vi "UDP Send and Receive (repeat on error) - DBL.vi"(7 "timeout ms (100)":i32=100, 8 "error in (no error)":errorcluster, 9 "DBL Command & Param":T1, 10 "IP":string, 11 "connection ID in":refnum<k16>) -> (0 "error out":errorcluster, 2 "DBL Param out":dbl, 3 "connection ID out":refnum<k16>)   [LabVIEW 2016, in "SMD-7615.lvlib" / "eSCL.lvlib"]
doc: "AC - Acceleration Rate\nSets or requests the acceleration rate used in point-to-point move commands in rev/sec/sec."
uses:
  eSCL.lvlib
  DBL Command and Param.ctl
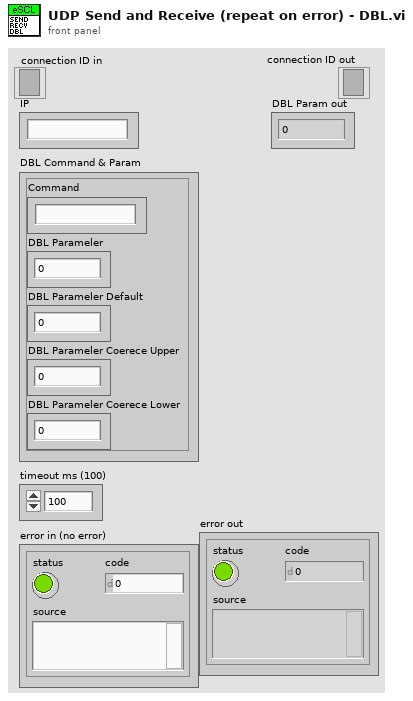
[diagram p1: front panel]
types:
  T1 = typedef "SMD-7615.lvlib/eSCL.lvlib/DBL Command and Param.ctl" = cluster{"Command":string, "DBL Parameler":dbl, "DBL Parameler Default":dbl, "DBL Parameler Coerece Upper":dbl, "DBL Parameler Coerece Lower":dbl}
  T2 = typedef "SMD-7615.lvlib/eSCL.lvlib/UDP Received Data.ctl" = cluster{"Received String":string, "eSCL Cmd":string, "Data":string}
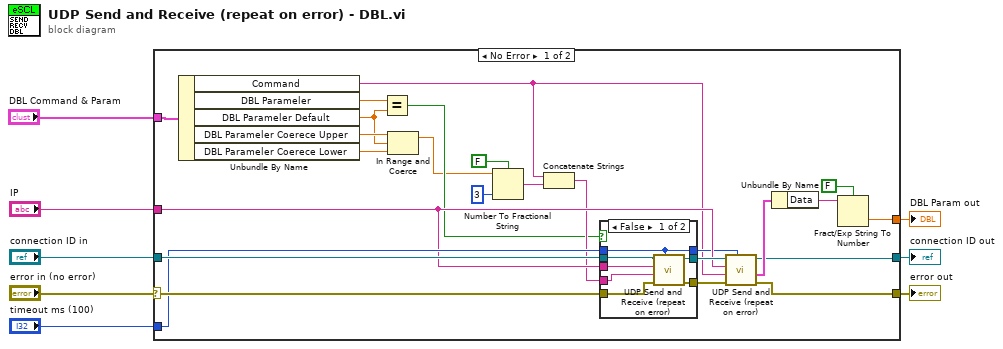
[diagram p0: block diagram]
diagram:
  n1 = case shown="No Error" "error in (no error)" {
    selector: "error in (no error)" -> [w33 w44]
    tunnel: "connection ID in" -> [w32 w45]
    tunnel: [w20 w45] -> w6
    tunnel: [w19 w44] -> w5
    tunnel: "IP" -> [w22 _]
    tunnel: "timeout ms (100)" -> [w23 _]
    tunnel: [w30 _] -> w2
    tunnel: "DBL Command & Param" -> [w14 _]
    frame No Error {
      n2 = Unbundle By Name(w14) -> ("Command"=w9:string, "DBL Parameler"=w13:dbl, "DBL Parameler Default"=w10:dbl, "DBL Parameler Coerece Upper"=w12:dbl, "DBL Parameler Coerece Lower"=w11:dbl)
      n3 = Equal?(x=w13, y=w10) -> (x = y?=w16:bool)
      n4 = In Range and Coerce(upper limit=w12, x=w10, lower limit=w11) -> (coerced(x)=w15:dbl)  [unwired: 1 out]
      n5 = Number To Fractional String(use system decimal point (T)=FALSE, number=w15, precision (6)=i16 3) -> (F-format string=w26:string)  [unwired: 1 in]
      n6 = Concatenate Strings(w9, w26) -> (w18:string)
      n7 = case shown="False" w16 {
        tunnel: w33 -> [w40 w41]
        tunnel: w32 -> [w39 w43]
        tunnel: [w38 w41] -> w25
        tunnel: [w37 w43] -> w24
        tunnel: w23 -> [w34 w42]
        tunnel: w22 -> [w36 _]
        tunnel: w18 -> [w35 _]
        tunnel: [w34 w42] -> w17
        frame False {
          n8 = call "UDP Send and Receive (repeat on error).vi"("timeout ms (100)"=w34, "error in (no error)"=w40, "Data"=w35, "IP"=w36, "connection ID in"=w39) -> ("error out"=w38:errorcluster, "connection ID out"=w37:refnum<k16>)  [unwired: 3 in, 2 out]
        }
        frame True {
        }
      }
      n9 = call "UDP Send and Receive (repeat on error).vi"("timeout ms (100)"=w17, "error in (no error)"=w25, "Data"=w9, "IP"=w22, "connection ID in"=w24) -> ("error out"=w19:errorcluster, "Received Data"=w21:T2, "connection ID out"=w20:refnum<k16>)  [unwired: 3 in, 1 out]
      n10 = Unbundle By Name(w21) -> ("Data"=w29:string)
      n11 = Fract/Exp String To Number(use system decimal point (T)=FALSE, string=w29) -> (number=w30:dbl)  [unwired: 2 in, 1 out]
    }
    frame Error {
    }
  }
  "connection ID out" <- w6
  "error out" <- w5
  "DBL Param out" <- w2
